vi "F43.vi"(8 "error in (no error)":errorcluster, 9 "data":u8[](array[numeric]), 10 "function":u8, 11 "device data model in":refnum<class "Standard Data Model.lvclass">) -> (0 "error out":errorcluster, 1 "data return":u8[](array[numeric]), 2 "function return":u8, 3 "device data model out":refnum<class "Standard Data Model.lvclass">)   [LabVIEW 2020, in "SubVIs.lvlib" / "Standard Data Model.lvclass"]
doc: "Executes function code 43"
uses:
  <vilib>/Modbus/subvis/Data and Functions/Standard Data Model/Standard Data Model.lvclass
  <vilib>/Modbus/subvis/Data and Functions/Device Data Model/Device Data Model.lvclass
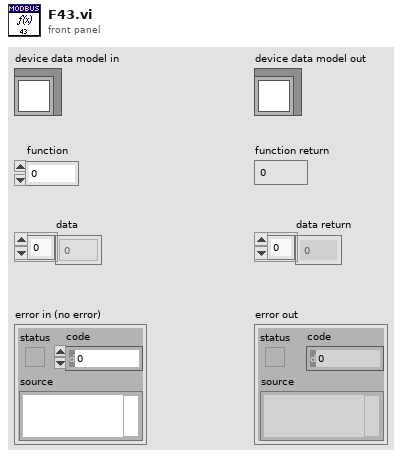
[diagram p1: front panel]
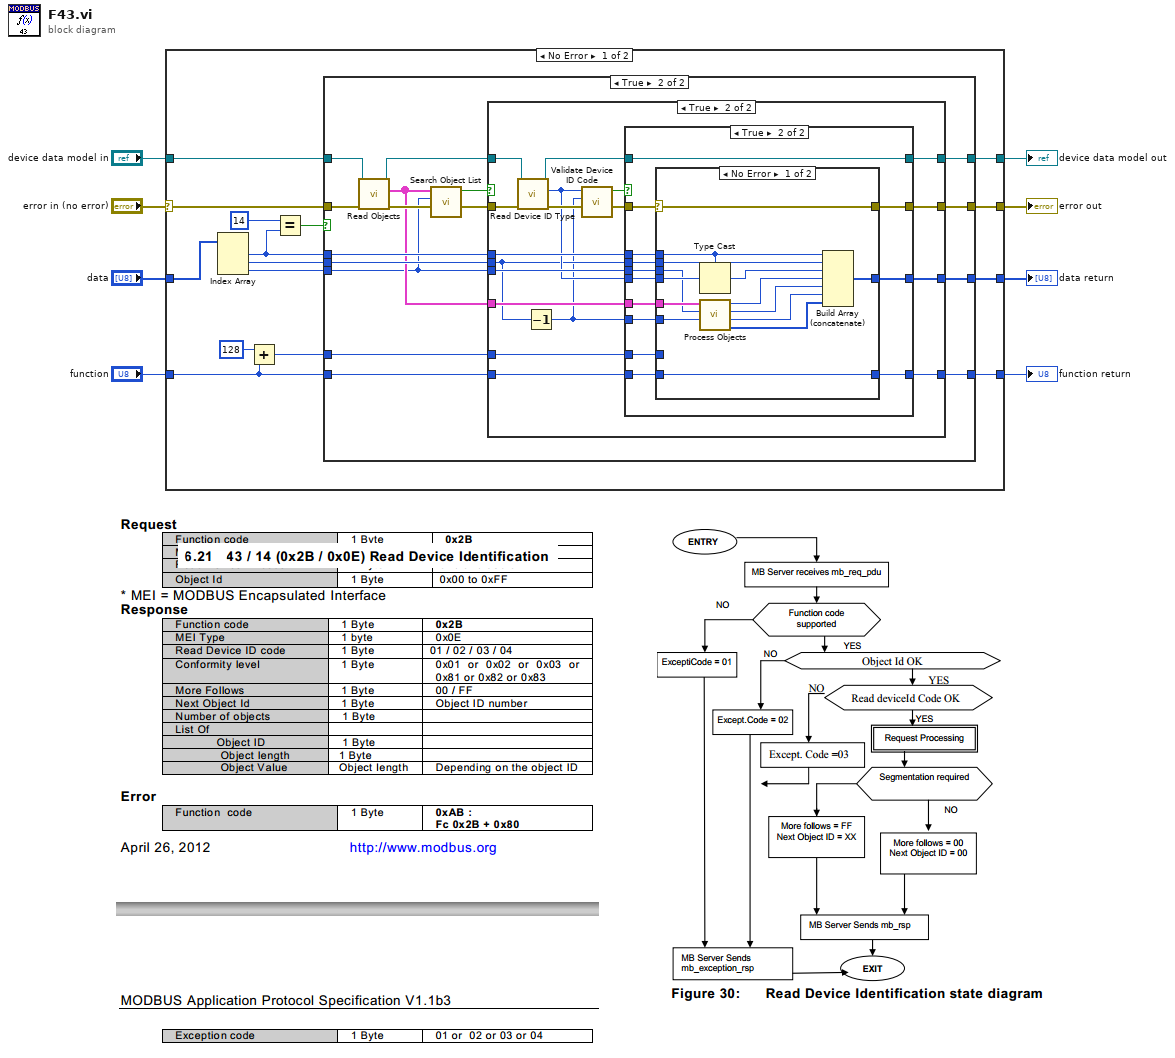
[diagram p0: block diagram]
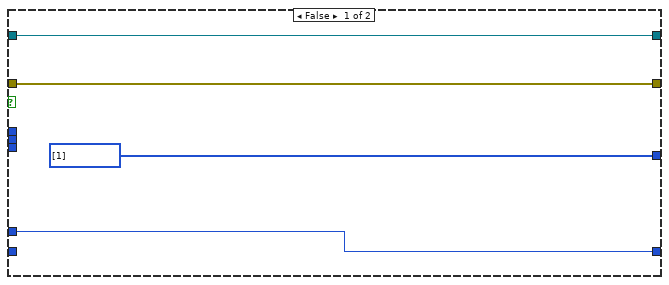
[diagram p2: hidden frame]
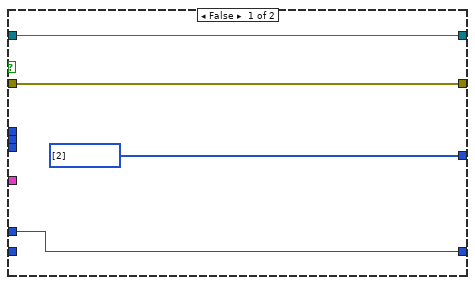
[diagram p3: hidden frame]
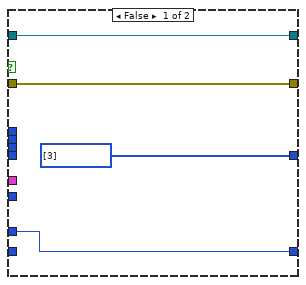
[diagram p4: hidden frame]
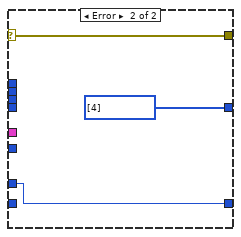
[diagram p5: hidden frame]
diagram:
  n1 = case shown="No Error" "error in (no error)" {
    selector: "error in (no error)" -> [w10 w101]
    tunnel: [w9 w101] -> w7
    tunnel: [w23 w100] -> w5
    tunnel: "device data model in" -> [w22 w100]
    tunnel: "function" -> [w19 w99]
    tunnel: "data" -> [w14 w98]
    tunnel: [w18 w99] -> w2
    tunnel: [w17 w98] -> w1
    frame No Error {
      n2 = Index Array(array=w14) -> (element #1=w11:u8, element #2=w16:u8, element #3=w15:u8)  [unwired: 3 in]
      n3 = Add(x=u8 128, y=w19) -> (x+y=w20:u8)
      n4 = Equal?(x=u8 14, y=w11) -> (x = y?=w12:bool)
      n5 = case shown="True" w12 {
        tunnel: [w27 w36] -> w23
        tunnel: w22 -> [w27 w42]
        tunnel: w20 -> [w26 w39]
        tunnel: w19 -> [_ w38]
        tunnel: [w26 w37] -> w18
        tunnel: [u8[] [1] ("Data Return") w40] -> w17
        tunnel: w16 -> [_ w33]
        tunnel: w15 -> [_ w30]
        tunnel: w11 -> [_ w32]
        tunnel: w10 -> [w24 w41]
        tunnel: [w24 w28] -> w9
        frame False {
        }
        frame True {
          n6 = call-dynamic "Read Objects.vi"("error in (no error)"=w41, "device data model in"=w42) -> ("error out"=w34:errorcluster, "objects"=w31:cluster{"object ID":u8, "value":string}[], "device data model out"=w35:refnum<class "Standard Data Model.lvclass">)  [unwired: 7 in]
          n7 = call <vilib>:"Search Object List.vi"("object ID"=w30, "objects"=w31) -> ("found?"=w29:bool)  [unwired: 7 in, 2 out]
          n8 = case shown="True" w29 {
            tunnel: [u8[] [2] ("Data Return") w57] -> w40
            tunnel: w39 -> [w45 w56]
            tunnel: w38 -> [_ w54]
            tunnel: [w45 w55] -> w37
            tunnel: [w44 w59] -> w36
            tunnel: w35 -> [w44 w63]
            tunnel: w34 -> [w43 w62]
            tunnel: w31 -> [_ w50]
            tunnel: w33 -> [_ w48]
            tunnel: w30 -> [_ w51]
            tunnel: w32 -> [_ w52]
            tunnel: [w43 w53] -> w28
            frame False {
            }
            frame True {
              n9 = call-dynamic "Read Device ID Type.vi"("error in (no error)"=w62, "device data model in"=w63) -> ("error out"=w58:errorcluster, "read device ID code"=w49:u8, "device data model out"=w60:refnum<class "Standard Data Model.lvclass">)  [unwired: 7 in]
              n10 = Decrement(x=w48) -> (x-1=w47:u8)
              n11 = call <vilib>:"Validate Device ID Code.vi"("read device ID code"=w47, "deivce conformity level"=w49) -> ("valid?"=w61:bool)  [unwired: 9 in]
              n12 = case shown="True" w61 {
                tunnel: w60 -> [w67 w80]
                tunnel: [w67 w80] -> w59
                tunnel: w58 -> [w64 w79]
                tunnel: [u8[] [3] ("Data Return") w78] -> w57
                tunnel: w56 -> [w65 w76]
                tunnel: [w65 w75] -> w55
                tunnel: w54 -> [_ w77]
                tunnel: [w64 w74] -> w53
                tunnel: w52 -> [_ w73]
                tunnel: w48 -> [_ w72]
                tunnel: w51 -> [_ w71]
                tunnel: w50 -> [_ w70]
                tunnel: w49 -> [_ w69]
                tunnel: w47 -> [_ w68]
                frame False {
                }
                frame True {
                  n13 = case shown="No Error" w79 {
                    selector: w79 -> [w94 w95]
                    tunnel: [w89 u8[] [4] ("Data Return")] -> w78
                    tunnel: w77 -> [w93 _]
                    tunnel: w76 -> [_ w96]
                    tunnel: [w93 w96] -> w75
                    tunnel: [w94 w95] -> w74
                    tunnel: w73 -> [w92 _]
                    tunnel: w72 -> [w82 _]
                    tunnel: w71 -> [w83 _]
                    tunnel: w70 -> [w88 _]
                    tunnel: w69 -> [w90 _]
                    tunnel: w68 -> [w81 _]
                    frame No Error {
                      n14 = Type Cast(type=w92, x=w90) -> (*(type *) &x=w91:u8)
                      n15 = call <vilib>:"Process Objects.vi"("read device ID code"=w81, "object ID"=w83, "objects"=w88) -> ("object data"=w84:u8[], "object count"=w85:u8, "next object ID"=w86:u8, "more follows"=w87:u8)  [unwired: 5 in]
                      n16 = Build Array (concatenate)(w92, w82, w91, w87, w86, w85, w84) -> (w89:u8[])
                    }
                    frame Error {
                    }
                  }
                }
              }
            }
          }
        }
      }
    }
    frame Error {
    }
  }
  "error out" <- w7
  "device data model out" <- w5
  "data return" <- w1
  "function return" <- w2
